vi "Set Scrollbars.vi"(8 "error in":errorcluster, 11 "Philips Subpanel in":refnum<class "Flex UI Subpanel.lvclass">) -> (0 "error out":errorcluster, 3 "Philips Subpanel out":refnum<class "Flex UI Subpanel.lvclass">)   [LabVIEW 2014, in "Flex UI Subpanel.lvclass"]
uses:
  Flex UI Subpanel.lvclass
  Flex UI (Parent)/Flex UI.lvclass/Flex UI.ctl
  Flex UI Subpanel.lvclass/Flex UI Subpanel.ctl
  Flex UI (Parent)/Flex UI.lvclass
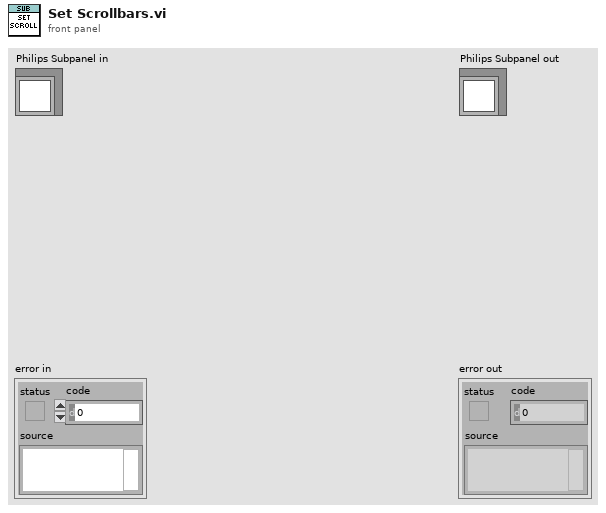
[diagram p1: front panel]
types:
  T1 = enum16{"Always On", "Always Off", "Off While Running"}
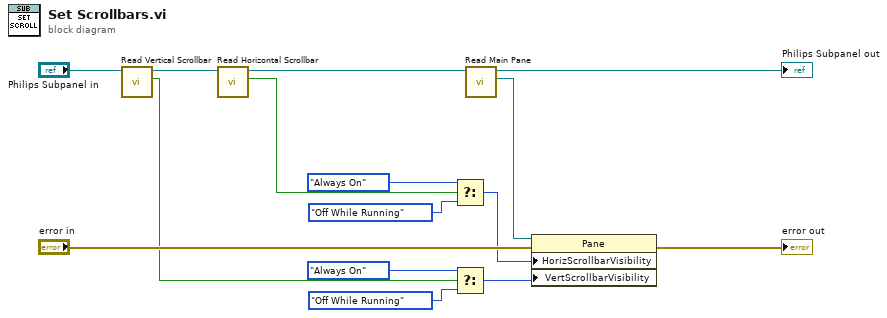
[diagram p0: block diagram]
diagram:
  n1 = call "Read Vertical Scrollbar.vi"("Philips Subpanel in"="Philips Subpanel in") -> ("Vertical Scrollbar"=w2:bool, "Philips Subpanel out"=w11:refnum<class "Flex UI Subpanel.lvclass">)  [unwired: 9 in]
  n2 = call "Read Horizontal Scrollbar.vi"("Philips Subpanel in"=w11) -> ("Horizontal Scrollbar"=w8:bool, "Philips Subpanel out"=w13:refnum<class "Flex UI Subpanel.lvclass">)  [unwired: 9 in]
  n3 = Select(t=T1."Always On" ("Horizontal Scrollbar Visibility"), s=w8, f=T1."Off While Running" ("Horizontal Scrollbar Visibility")) -> (s? t:f=w5:T1)
  n4 = Select(t=T1."Always On" ("Horizontal Scrollbar Visibility"), s=w2, f=T1."Off While Running" ("Horizontal Scrollbar Visibility")) -> (s? t:f=w1:T1)
  n5 = call "Read Main Pane.vi"("Philips UI in"=w13) -> ("Main Pane"=w9:refnum<vi>, "Philips UI out"=→"Philips Subpanel out":refnum<class "Flex UI Subpanel.lvclass">)  [unwired: 9 in]
  n6 = property class="Pane"(reference=w9, error in="error in", "HorizScrollbarVisibility"=w5, "VertScrollbarVisibility"=w1) -> (error out=→"error out":errorcluster)  [unwired: 1 out]
